vi "Initialize.vi"(8 "error in":errorcluster, 9 "parameters":variant, 10 "path":path, 11 "repository in":refnum<class "NISE_CEF_HierarchyRepo.lvclass">) -> (0 "error out":errorcluster, 3 "repository out":refnum<class "NISE_CEF_HierarchyRepo.lvclass">)   [LabVIEW 2013, in "NISE_CEF_HierarchyRepo.lvclass"]
doc: "Initializes the repo. StoreClassPath method should be called in this VI"
uses:
  NISE_CEF_HierarchyRepo.lvclass
  Repository/NISE_CEF_Repository.lvclass
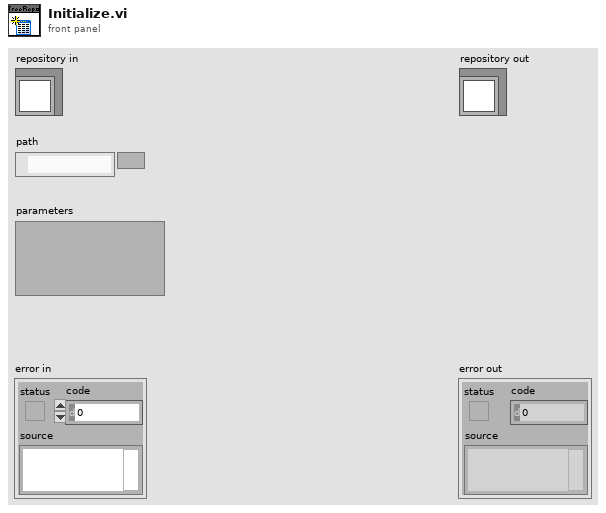
[diagram p1: front panel]
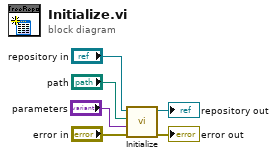
[diagram p0: block diagram]
diagram:
  n1 = call-parent "Initialize.vi"("error in"="error in", "parameters"="parameters", "path"="path", "repository in"="repository in") -> ("error out"=→"error out":errorcluster, "repository out"=→"repository out":refnum<class "NISE_CEF_HierarchyRepo.lvclass">)  [unwired: 6 in]
